vi "Power High_Low Control.vi"(0 "Resource Name":string="GPIB0::1::INSTR", 5 "error in (no error)":errorcluster, 6 "Output":bool, 9 "Voltage":dbl format="%^.2e") -> (14 "Instrument Handle out":refnum<k15>, 16 "Output":string, 19 "error out":errorcluster)   [LabVIEW 2014]
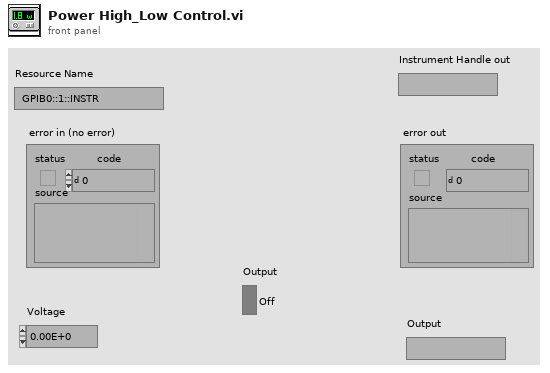
[diagram p1: front panel]
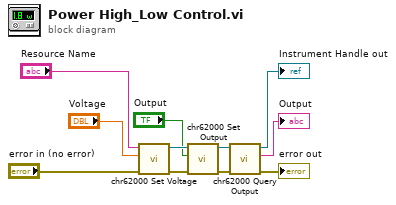
[diagram p0: block diagram]
diagram:
  n1 = call "chr62000 Set Voltage.vi"("error in (no error)"="error in (no error)", "Voltage"="Voltage", "Instrument Handle"="Resource Name") -> ("error out"=w10:errorcluster, "Instrument Handle out"=w9:refnum<k15>)  [unwired: 7 in]
  n2 = call "chr62000 Set Output.vi"("error in (no error)"=w10, "Output"="Output", "Instrument Handle"=w9) -> ("error out"=w6:errorcluster, "Instrument Handle out"=w7:refnum<k15>)  [unwired: 7 in]
  n3 = call "chr62000 Query Output.vi"("error in (no error)"=w6, "Instrument Handle"=w7) -> ("error out"=→"error out":errorcluster, "Output"=→"Output":string, "Instrument Handle out"=→"Instrument Handle out":refnum<k15>)  [unwired: 7 in]
